vi "Inverse Chirp Z Transform.vi"(8 "increment":cdb=1.0+0.1i, 9 "starting point":cdb=1.0+0.0i, 10 "# of samples":i32=-1, 11 "Chirp-Z {X}":cdb[](array[numeric])) -> (0 "error":i32, 3 "X":cdb[](array[numeric]))   [LabVIEW 2020, in "NI_AALPro.lvlib"]
doc: "Computes the inverse Chirp-Z transform of the input sequence <B>Chirp-Z {X}</B>."
uses:
  <vilib>/Analysis/NI_AALPro.lvlib
  <resource>/lvanlys.dll
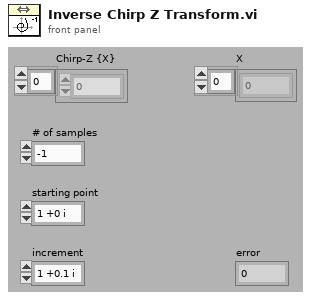
[diagram p1: front panel]
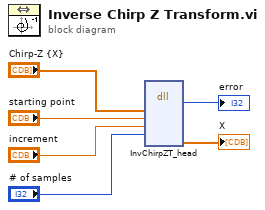
[diagram p0: block diagram]
diagram:
  n1 = dll-call lib="e:/builds/penguin/labview/branches/2020/dev/dist/resource/lvanlys.*" fn="InvChirpZT_head"("Chirp-Z {X}"="Chirp-Z {X}", "starting point"="starting point", "increment"="increment", "n"="# of samples") -> (→"error":i32, "X"=→"X":cdb[])  [unwired: 8 in, 2 out]
